vi "_get_float4.vi"(7 "错误输入（无错误）":errorcluster, 8 "写入缓冲区":string, 9 "连接ID":refnum<k5>) -> (0 "错误输出":errorcluster, 1 "值 3":sgl, 2 "值 2":sgl, 3 "值":sgl, 4 "值 4":sgl, 5 "连接ID输出":refnum<k5>)   [LabVIEW 2017]
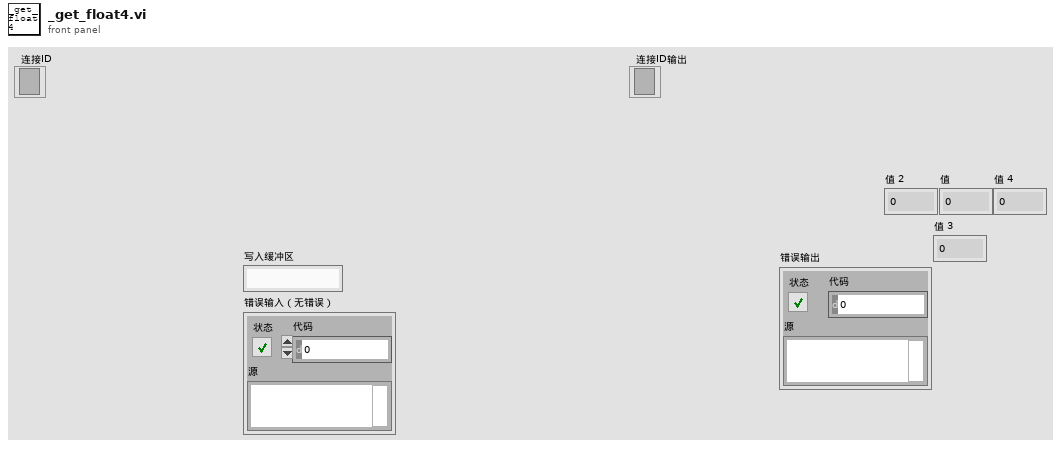
[diagram p1: front panel]
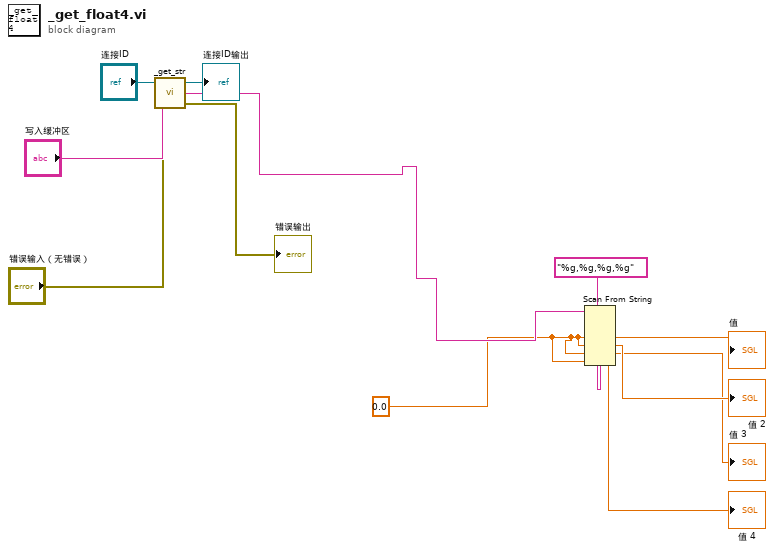
[diagram p0: block diagram]
diagram:
  w3 = sgl 0.0 ("默认值 1")
  n1 = call "_get_str.vi"("错误输入（无错误）"="错误输入（无错误）", "写入缓冲区"="写入缓冲区", "连接ID"="连接ID") -> ("错误输出"=→"错误输出":errorcluster, "读取缓冲区"=w9:string, "连接ID输出"=→"连接ID输出":refnum<k5>)
  n2 = Scan From String(format string="%g,%g,%g,%g" ("格式字符串"), input string=w9, default 1=w3, default 2=w3, default 3=w3, default 4=w3) -> (output 1=→"值":sgl, output 2=→"值 2":sgl, output 3=→"值 3":sgl, output 4=→"值 4":sgl)  [unwired: 2 in, 3 out]
